vi "Save.vi"(8 "error in":errorcluster, 11 "state in":T1) -> (0 "error out":errorcluster, 3 "state out":T1)   [LabVIEW 2014, in "CI Project Builder.lvlib"]
doc: "This VI calls the Repo Save VI passing the current Path. Updating the unsaved changes flag if the save is succesfull."
uses:
  CI Project Builder.lvlib
  Controls/StateCluster.ctl
  <vilib>/ni/Configuration Framework/Node/NodeRef.ctl
  <vilib>/ni/Configuration Framework/Node/NISE_CEF_Node.lvclass
  <vilib>/ni/Configuration Framework/Node/StandardEvents.ctl
  <vilib>/ni/Configuration Framework/Node/UserEventRef.ctl
  <vilib>/ni/Configuration Framework/Controls/EventCluster.ctl
  <vilib>/ni/Configuration Framework/Node/NodeChangeEvent.ctl
  <vilib>/ni/Configuration Framework/Node/CacheState.ctl
  <vilib>/ni/Configuration Framework/Node/RefreshUIEvent.ctl
  <vilib>/ni/Configuration Framework/Node/StopEvent.ctl
  <vilib>/ni/Configuration Framework/glyph manager/glyph manager.ctl
  <vilib>/picture/picture.llb/imagedata.ctl
  Classes/INI Serializer/INI Serializer.lvclass
  Classes/CI Serializer/CI Serializer.lvclass
  <vilib>/ni/Configuration Framework/NISE_CEF_TreeControl.lvlib
  <vilib>/ni/Configuration Framework/glyph manager/glyph manager.lvlib
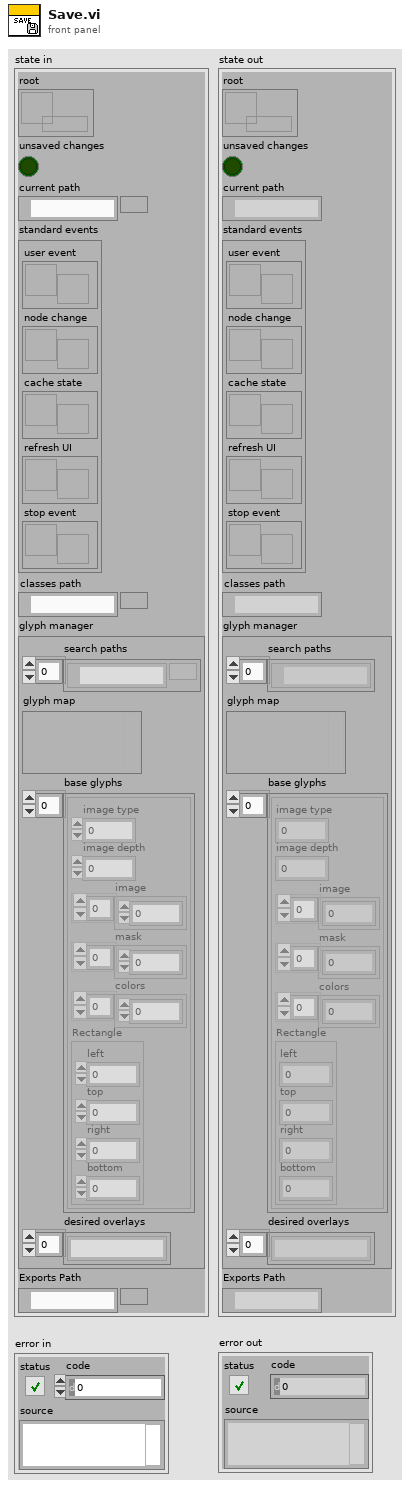
[diagram p1: front panel]
types:
  T1 = typedef "CI Project Builder.lvlib/StateCluster.ctl" = cluster{"root":T2, "unsaved changes":bool, "current path":path, "standard events":T3, "classes path":path, "glyph manager":T9, "Exports Path":path}
  T2 = typedef "NISE_CEF_Node.lvclass/NodeRef.ctl" = refnum<data-value>
  T3 = typedef "NISE_CEF_Node.lvclass/StandardEvents.ctl" = cluster{"user event":T4, "node change":T5, "cache state":T6, "refresh UI":T7, "stop event":T8}
  T4 = typedef "NISE_CEF_Node.lvclass/UserEventRef.ctl" = refnum<user-event>
  T5 = typedef "NISE_CEF_Node.lvclass/NodeChangeEvent.ctl" = refnum<user-event>
  T6 = typedef "NISE_CEF_Node.lvclass/CacheState.ctl" = refnum<user-event>
  T7 = typedef "NISE_CEF_Node.lvclass/RefreshUIEvent.ctl" = refnum<user-event>
  T8 = typedef "NISE_CEF_Node.lvclass/StopEvent.ctl" = refnum<user-event>
  T9 = typedef "glyph manager.lvlib/glyph manager.ctl" = cluster{"search paths":path[], "glyph map":variant, "base glyphs":T10[], "desired overlays":string[]}
  T10 = typedef "imagedata.ctl" = cluster{"image type":i32, "image depth":i32, "image":u8[], "mask":u8[], "colors":u32[], "Rectangle":cluster{"left":i16, "top":i16, "right":i16, "bottom":i16}}
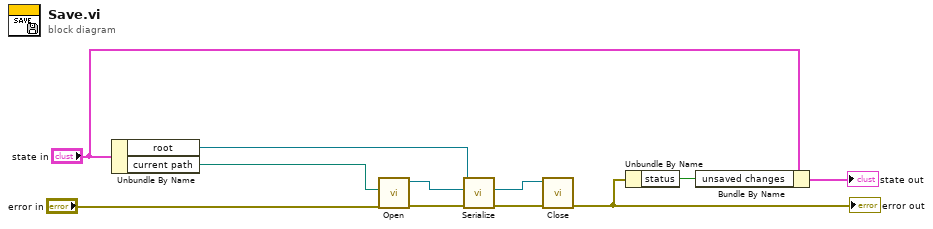
[diagram p0: block diagram]
diagram:
  n1 = Unbundle By Name("state in") -> ("root"=w1:T2, "current path"=w2:path)
  n2 = call "Open.vi"("error in (no error)"="error in", "INI Path"=w2) -> ("error out"=w8:errorcluster, "INI Serializer out"=w7:refnum<class "INI Serializer.lvclass">)  [unwired: 8 in]
  n3 = call "Serialize.vi"("error in (no error)"=w8, "CI Serializer in"=w7, "Root Node"=w1) -> ("error out"=w5:errorcluster, "CI Serializer out"=w6:refnum<class "INI Serializer.lvclass">)  [unwired: 7 in]
  n4 = call "Close.vi"("error in (no error)"=w5, "INI Serializer in"=w6) -> ("error out"=w4:errorcluster)  [unwired: 9 in]
  "error out" <- w4
  n5 = Unbundle By Name(w4) -> ("status"=w9:bool)
  n6 = Bundle By Name(cluster="state in", "unsaved changes"=w9) -> (→"state out":T1)
